vi "Main.vi"() -> ()   [LabVIEW 2020]
doc: "Este vi sirve para el control de monturas mecánicas y adquisición de datos de 2 instrumentos físicos.\n\nSolicitante:\nDr. Gabriel Ramos"
uses:
  <instrlib>/ZaberTSeries/Public/Utility/Request.ctl
  <instrlib>/ZaberTSeries/ZaberTSeries.lvlib
  Type Definitions/Datos a Guardar.ctl
  <vilib>/Utility/error.llb/DialogType.ctl
  <instrlib>/ZaberTSeries/Public/Utility/Response.ctl
  Type Definitions/Asistente de adquisicion Cluster.ctl
  <instrlib>/Stanford Research 830/Stanford Research 830.lvlib
  <instrlib>/Tektronix TDS 200 1000 2000 Series/Tektronix TDS 200 1000 2000 Series.lvlib
  Type Definitions/datos osciloscopio.ctl
  Type Definitions/Datos Zaber.ctl
  Type Definitions/parametros motores.ctl
  <instrlib>/Control de MaP/Control de MaP.lvlib
panel:
  out "Posición Actual":dbl[unit](slide) max=0.05
  in  "Stop Button":bool
  out "Datos":dbl[](graph)
  out "stop":bool
  out "Datos actuales":T1
  # "ENA"
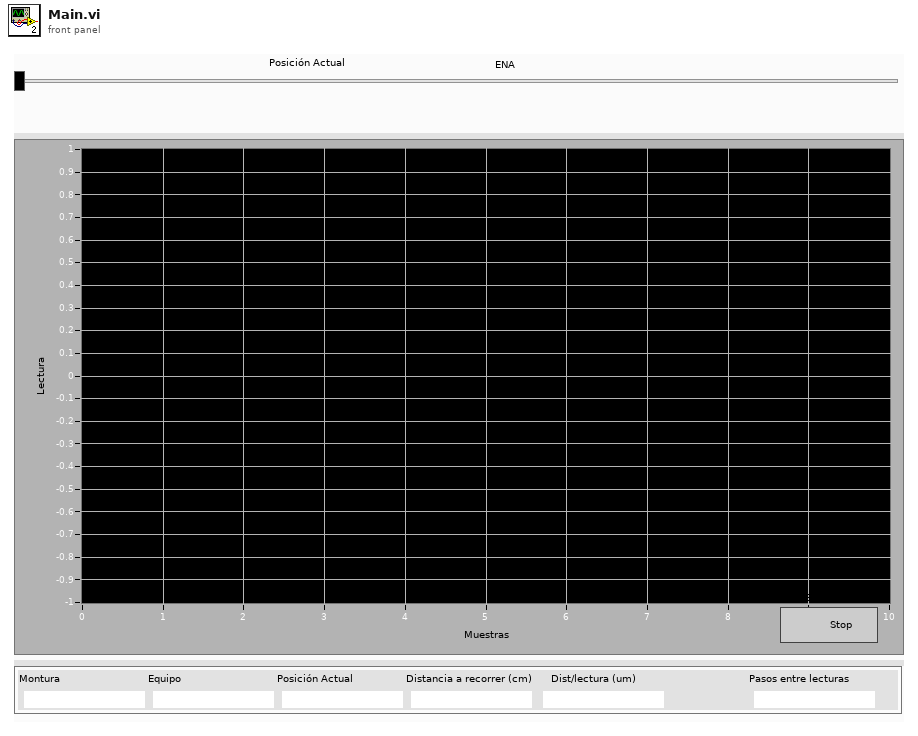
[diagram p1: front panel]
types:
  T1 = cluster{"Montura":string, "Equipo":string, "Posición Actual":string, "Distancia a recorrer (cm)":string, "Dist/lectura (um)":string, "Pasos entre lecturas":string}
  T2 = typedef "Asistente de adquisicion Cluster.ctl" = cluster{"Montura":enum16{"Zaber T-LSR450B", "Motor Bipolar", "Motor Unipolar"}, "Equipo a Utilizar":enum16{"SR830 Lock In", "TDS 2012B Osciloscope"}, "Datos Zaber":T3, "Datos Bipolar/Unipolar":T4, "Datos Archivo":cluster{"Ruta Archivo":path, "Nombre de Prueba":string}, "Datos actuales":cluster{"Montura":string, "Equipo":string, "Posición Actual":string, "Distancia Total a recorrer":string, "distancia Entre lecturas":string, "Pasos entre lecturas":string}, "Datos a Guardar In":T5, "Datos Osciloscopio":T6, "Datos Lock In":cluster{"Visa Lock in":refnum<visa-resource-name>}}
  T3 = typedef "Datos Zaber.ctl" = cluster{"Sentido de Adquisición":bool, "Comenzar Desde Home?":bool, "Distancia a recorrer (cm)":dbl, "Pasos motor":i32, "Distancia entre Lecturas (um)":dbl, "Puerto":refnum<visa-resource-name>}
  T4 = typedef "parametros motores.ctl" = cluster{"Puerto COM":refnum<visa-resource-name>, "Pasos entre Lecturas":u16, "Numero de lecturas":u32, "Sentido del motor":bool}
  T5 = typedef "Datos a Guardar.ctl" = cluster{"Datos Cursor Tektronix":string, "Datos Lokin":string, "Posición Cero":dbl[unit], "Posición Actual":dbl[unit]}
  T6 = typedef "datos osciloscopio.ctl" = cluster{"Sesión Visa Osciloscopio":refnum<visa-resource-name>, "Tipo de Adquisición":enum16{"Voltaje Pico Pico", "Voltaje RMS", "Cursor Tiempo"}, "Canal a Utilizar":enum16{"Canal 1", "Canal 2", "Canal 1 y 2"}, "Parametros de Adquisición":enum16{"Una Muestra", "Promedio"}, "Número Promedio":i32}
  T7 = typedef "ZaberTSeries.lvlib/Response.ctl" = cluster{"Device Number":u8, "Command":u8, "Data":i32}
  T8 = typedef "DialogType.ctl" = u16
  T9 = typedef "Constante estados proceso adquisición.ctl" = enum16{"Inicializar Equipo", "Inicializar Montura", "Leer Pos Actual", "Inicializar Archivo", "Leer Equipo", "guardar Archivo", "Mover Montura", "Corroborar distancias y Stop", "Cerrar Archivo y equipos"}
  T10 = typedef "ZaberTSeries.lvlib/Request.ctl" = cluster{"Device Number":u8, "Command":u8, "Data":i32, "Response Count":i32}
  T11 = enum16{"Zaber T-LSR450B", "Motor Bipolar", "Motor Unipolar"}
  T12 = cluster{"Montura":string, "Equipo":string, "Posición Actual":string, "Distancia Total a recorrer":string, "distancia Entre lecturas":string, "Pasos entre lecturas":string}
  T13 = enum32{"invalid app kind", "Development System", "Run Time System", "Student Edition", "Embedded LabVIEW", "Evaluation", "Custom"}
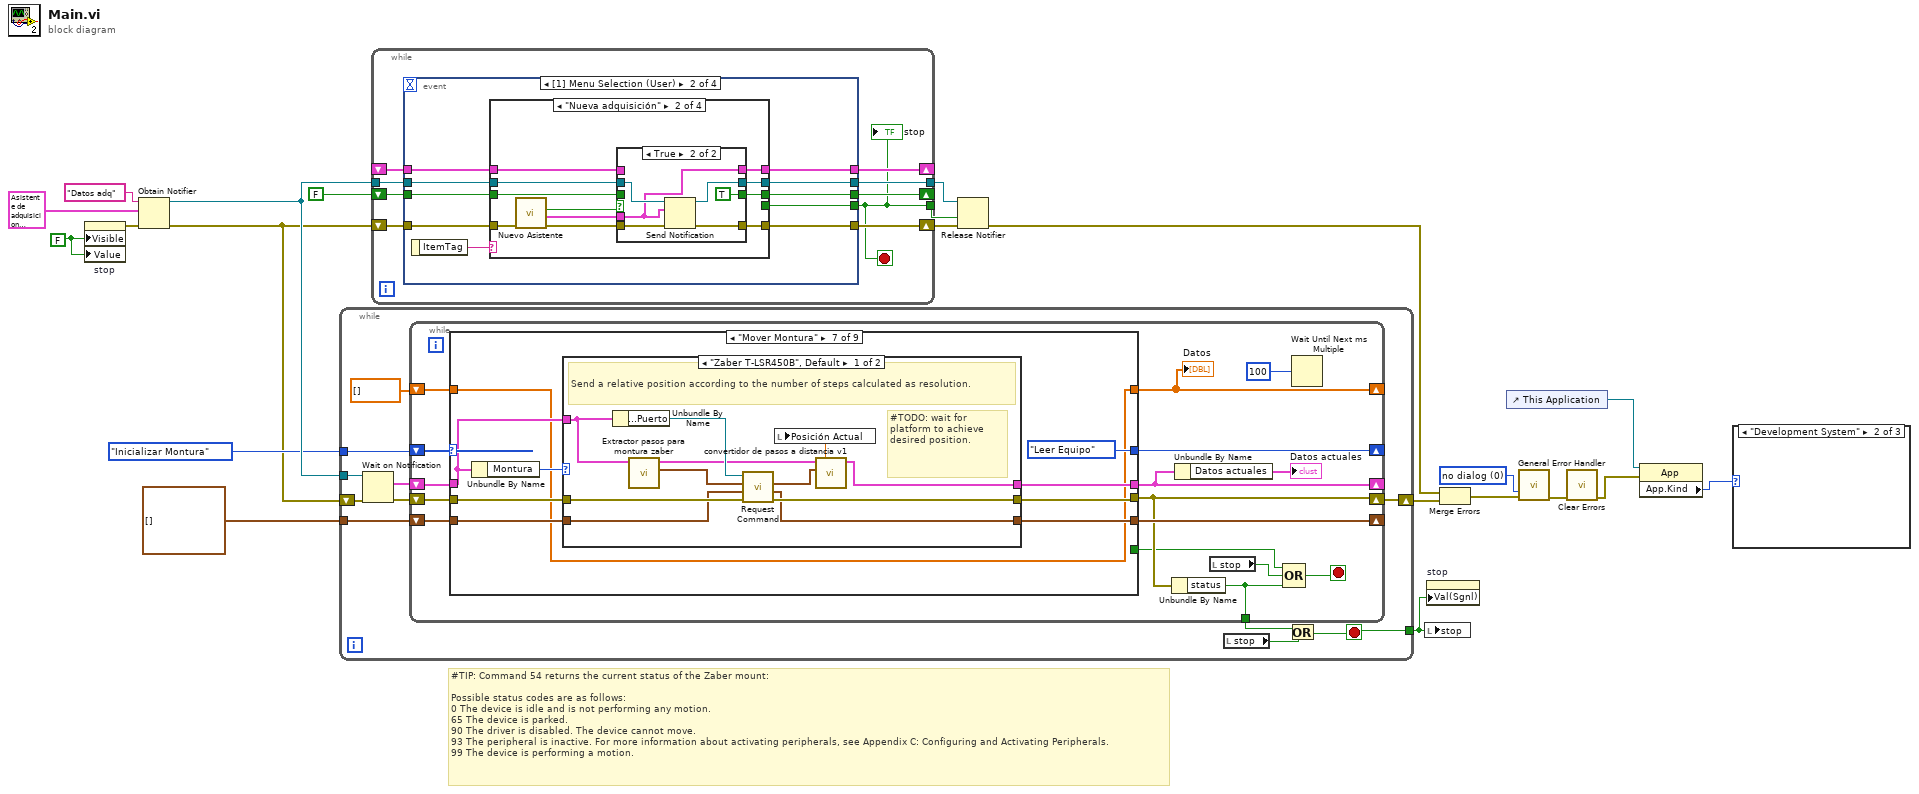
[diagram p0: block diagram]
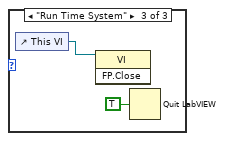
[diagram p3: hidden frame]
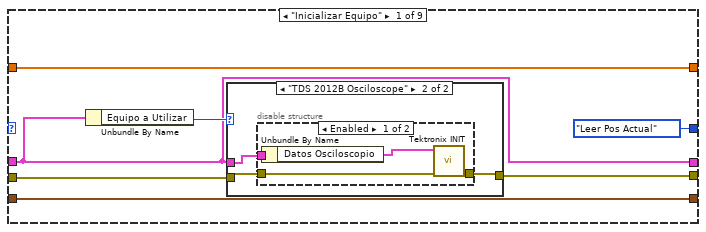
[diagram p4: hidden frame]
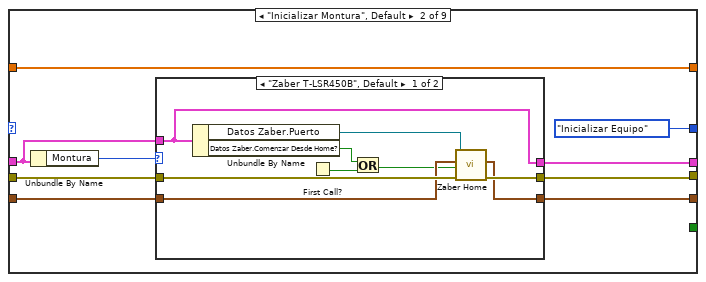
[diagram p7: hidden frame]
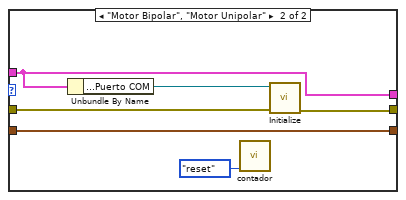
[diagram p8: hidden frame]
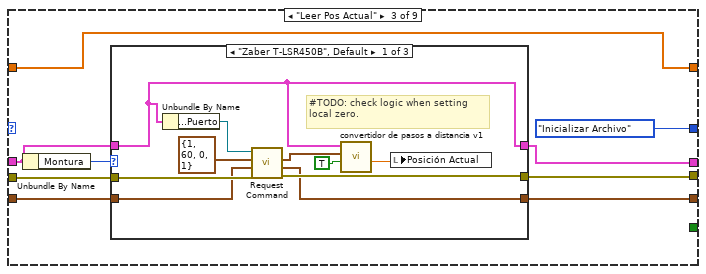
[diagram p9: hidden frame]
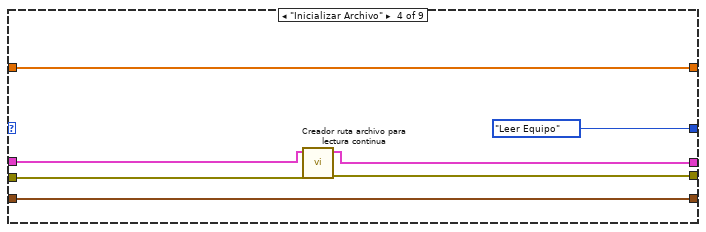
[diagram p12: hidden frame]
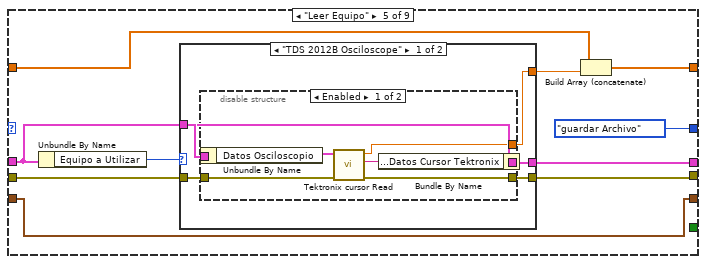
[diagram p13: hidden frame]
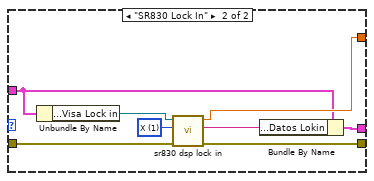
[diagram p15: hidden frame]
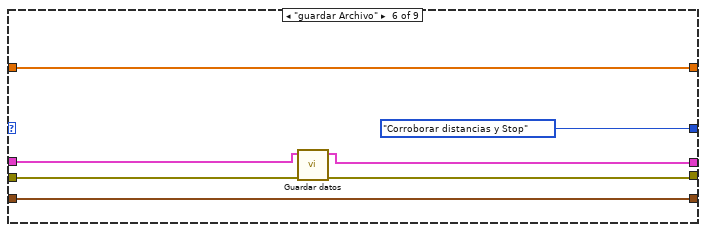
[diagram p16: hidden frame]
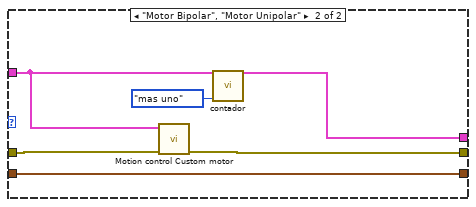
[diagram p17: hidden frame]
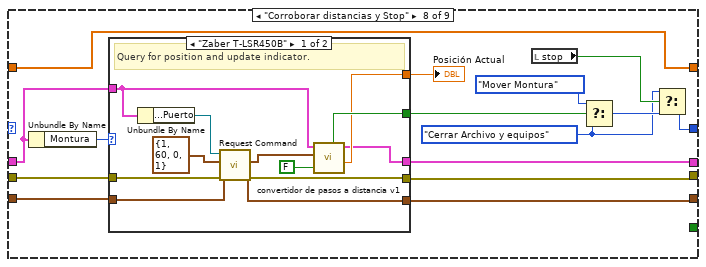
[diagram p18: hidden frame]
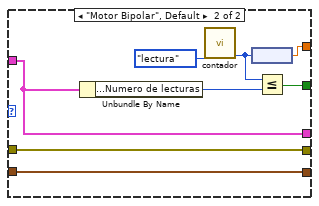
[diagram p19: hidden frame]
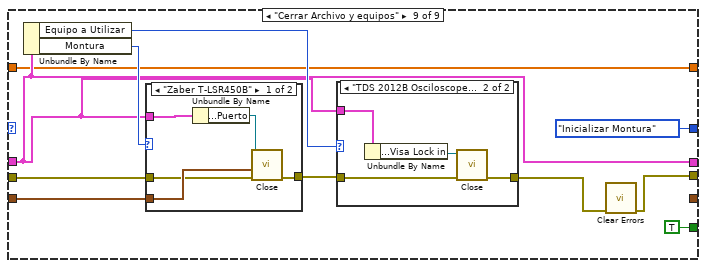
[diagram p20: hidden frame]
diagram:
  w2 = FALSE ("Visible")
  w12 = T8 0 items=["no dialog", "OK message", "continue or stop message", "OK message + warnings", "continue/stop + warnings"] ("type of dialog (OK msg:1)")
  # "#TIP: Command 54 returns the current status of the Zaber mount:\n\nPossible status codes are as follows:\n0 The device is idle and is not performing any motion.\n65 The device is parked.\n90 The driver is disabled. The device cannot move.\n93 The peripheral is inactive. For more information about activating peripherals, see Appendix C: Configuring and Activating Peripherals.\n99 The device is performing a motion."
  n1 = property on="stop" class="Bool (strict)"("Visible"=w2, "Value"=w2) -> (error out=w8:errorcluster)  [unwired: 2 in, 1 out]
  n2 = Obtain Notifier(name (unnamed)="Datos adq", notification data type=T2 {"Montura"=enum."Motor Bipolar", "Equipo a Utilizar"=enum."TDS 2012B Osciloscope", "Datos Zaber"={"Sentido de Adquisición"=FALSE, "Comenzar Desde Home?"=FALSE, "Distancia a recorrer (cm)"=0.0, "Pasos motor"=0, "Distancia entre Lecturas (um)"=0.0, "Puerto"=""}, "Datos Bipolar/Unipolar"={"Puerto COM"="", "Pasos entre Lecturas"=0, "Numero de lecturas"=0, "Sentido del motor"=TRUE}, "Datos Archivo"={"Ruta Archivo"=path "", "Nombre de Prueba"=""}, "Datos actuales"={"Montura"="", "Equipo"="", "Posición Actual"="", "Distancia Total a recorrer"="", "distancia Entre lecturas"="", "Pasos entre lecturas"=""}, "Datos a Guardar In"={"Datos Cursor Tektronix"="", "Datos Lokin"="", "Posición Cero"=0.0, "Posición Actual"=0.0}, "Datos Osciloscopio"={"Sesión Visa Osciloscopio"="Tektronix_TDS2012C", "Tipo de Adquisición"=enum."Voltaje Pico Pico", "Canal a Utilizar"=enum."Canal 1", "Parametros de Adquisición"=enum."Una Muestra", "Número Promedio"=2}, "Datos Lock In"={"Visa Lock in"="Tektronix_TDS2012C"}} ("Datos de Nueva Adquisición In"), error in (no error)=w8) -> (notifier out=w20:refnum<notifier>, error out=w11:errorcluster)  [unwired: 1 in, 1 out]
  n3 = while {
    tunnel: w20 -> [w32]
    shift-right: [w27] -> w15
    shift-left: w11 -> [w31]
    tunnel: Constante_estados_proceso_adquisición."Inicializar Montura" -> [w28]
    tunnel: T7[] [] ("Responses in") -> [w24]
    tunnel: [w23] -> w7
    stop <- w23 stop-if-true
    n4 = Wait on Notification(notifier=w32, error in (no error)=w31) -> (notification=w29:T2, error out=w30:errorcluster)  [unwired: 2 in, 2 out]
    n5 = while {
      shift-right: [w47] -> _
      shift-left: w28 -> [w48]
      shift-right: [w38] -> w27
      shift-left: w30 -> [w45]
      shift-right: [w39] -> _
      shift-left: w29 -> [w40]
      tunnel: [w35] -> w26
      shift-right: [w42] -> _
      shift-left: w24 -> [w43]
      shift-right: [w33] -> _
      shift-left: dbl[] [] -> [w34]
      stop <- w44 stop-if-true
      n6 = case shown="\"Mover Montura\"" w48 {
        tunnel: w40 -> [w52 w70 w93 w115 w127 w154 w164 w193 w224]
        tunnel: w45 -> [w51 w72 w96 w118 w129 w157 w166 w197 w226]
        tunnel: [w50 w71 w95 w117 w128 w156 w165 w196 w222] -> w38
        tunnel: [Constante_estados_proceso_adquisición."Leer Pos Actual" ("f") Constante_estados_proceso_adquisición."Inicializar Equipo" Constante_estados_proceso_adquisición."Inicializar Archivo" ("f") Constante_estados_proceso_adquisición."Leer Equipo" ("f") Constante_estados_proceso_adquisición."guardar Archivo" ("f") Constante_estados_proceso_adquisición."Corroborar distancias y Stop" ("f") Constante_estados_proceso_adquisición."Leer Equipo" ("f") w187 Constante_estados_proceso_adquisición."Inicializar Montura" ("f")] -> w47
        tunnel: [w52 w67 w90 w114 w124 w153 w161 w188 w224] -> w39
        tunnel: [_ _ _ _ _ _ _ _ TRUE ("stop")] -> w37
        tunnel: w43 -> [w49 w69 w92 w119 w125 w158 w163 w195 w227]
        tunnel: [w49 w68 w91 w119 w125 w158 w162 w194 _] -> w42
        tunnel: [w55 w66 w89 w116 w122 w155 w160 w186 w221] -> w33
        tunnel: w34 -> [w55 w66 w89 w116 w121 w155 w160 w186 w221]
        frame "Inicializar Equipo" {
          n7 = Unbundle By Name(w52) -> ("Equipo a Utilizar"=w53:enum16{"SR830 Lock In", "TDS 2012B Osciloscope"})
          n8 = case shown="\"TDS 2012B Osciloscope\"" w53 {
            tunnel: w52 -> [_ w59]
            tunnel: w51 -> [w56 w58]
            tunnel: [w56 w57] -> w50
            frame "SR830 Lock In", Default {
            }
            frame "TDS 2012B Osciloscope" {
              n9 = disable-structure shown="Enabled" {
                disable-tunnel: w59 -> [w63 _]
                disable-tunnel: w58 -> [w61 w64]
                disable-tunnel: [w60 w64] -> w57
                frame Enabled {
                  n10 = Unbundle By Name(w63) -> ("Datos Osciloscopio"=w62:T6)
                  n11 = call "Tektronix INIT.vi"("error in (no error)"=w61, "Datos Osciloscopio"=w62) -> ("error out"=w60:errorcluster)  [unwired: 9 in]
                }
                frame Disabled {
                }
              }
            }
          }
        }
        frame "Inicializar Montura", Default {
          n12 = Unbundle By Name(w70) -> ("Montura"=w73:T11)
          n13 = case shown="\"Zaber T-LSR450B\", Default" w73 {
            tunnel: w72 -> [w82 w86]
            tunnel: [w81 w85] -> w71
            tunnel: w70 -> [w78 w84]
            tunnel: w69 -> [w79 w88]
            tunnel: [w77 w88] -> w68
            tunnel: [w78 w84] -> w67
            frame "Zaber T-LSR450B", Default {
              n14 = Unbundle By Name(w78) -> ("Datos Zaber.Puerto"=w80:refnum<visa-resource-name>, "Datos Zaber.Comenzar Desde Home?"=w75:bool)
              n15 = First Call?() -> (First Call?: T/F=w76:bool)
              n16 = Or(x=w75, y=w76) -> (x .or. y?=w74:bool)
              n17 = call "Zaber Home.vi"("error in (no error)"=w82, "Ir a Home"=w74, "Responses in"=w79, "VISA Refnum in"=w80) -> ("error out"=w81:errorcluster, "Responses out"=w77:T7[])  [unwired: 5 in, 1 out]
            }
            frame "Motor Bipolar", "Motor Unipolar" {
              n18 = Unbundle By Name(w84) -> ("Datos Bipolar/Unipolar.Puerto COM"=w87:refnum<visa-resource-name>)
              n19 = call "contador.vi"("Opciones"=enum16{"reset", "mas uno", "lectura"}."reset") -> ()  [unwired: 10 in, 1 out]
              n20 = call <instrlib>:"Initialize.vi"("error in (no error)"=w86, "Puerto Serial"=w87) -> ("error out"=w85:errorcluster)  [unwired: 8 in, 1 out]
            }
          }
        }
        frame "Leer Pos Actual" {
          n21 = Unbundle By Name(w93) -> ("Montura"=w97:T11)
          n22 = case shown="\"Zaber T-LSR450B\", Default" w97 {
            tunnel: w96 -> [w107 w110 w113]
            tunnel: [w106 w110 w113] -> w95
            tunnel: w93 -> [w98 w108 w111]
            tunnel: w92 -> [w105 w109 w112]
            tunnel: [w104 w109 w112] -> w91
            tunnel: [w98 w108 w111] -> w90
            frame "Zaber T-LSR450B", Default {
              # "#TODO: check logic when setting local zero."
              n23 = Unbundle By Name(w98) -> ("Datos Zaber.Puerto"=w102:refnum<visa-resource-name>)
              n24 = call <instrlib>:"Request Command.vi"("error in (no error)"=w107, "Responses in"=w105, "Request"=T10 {"Device Number"=1, "Command"=60, "Data"=0, "Response Count"=1}, "VISA resource name"=w102) -> ("error out"=w106:errorcluster, "Responses out"=w104:T7[], "First Response"=w100:T7)  [unwired: 4 in, 1 out]
              n25 = call "convertidor de pasos a distancia v1.vi"("Set 0 vitual"=TRUE ("Inicializar"), "Respuesta Zaber"=w100, "Datos adquisición Input"=w98) -> ("Respuesta conversión zaber"=w103:dbl[unit])  [unwired: 6 in, 2 out]
              n26 = local write "Posición Actual"(w103) -> ()
            }
            frame "Motor Bipolar" {
            }
            frame "Motor Unipolar" {
            }
          }
        }
        frame "Inicializar Archivo" {
          n27 = call "Creador ruta archivo para lectura continua.vi"("error in (no error)"=w118, "Datos de Nueva Adquisición In"=w115) -> ("error out"=w117:errorcluster, "Datos de Nueva Adquisición out"=w114:T2)  [unwired: 4 in]
        }
        frame "Leer Equipo" {
          n28 = Unbundle By Name(w127) -> ("Equipo a Utilizar"=w130:enum16{"SR830 Lock In", "TDS 2012B Osciloscope"})
          n29 = case shown="\"TDS 2012B Osciloscope\"" w130 {
            tunnel: w127 -> [w133 w146]
            tunnel: w129 -> [w135 w151]
            tunnel: [w134 w150] -> w128
            tunnel: [w131 w147] -> w123
            tunnel: [w132 w145] -> w124
            frame "TDS 2012B Osciloscope" {
              n30 = disable-structure shown="Enabled" {
                disable-tunnel: w135 -> [w142 w143]
                disable-tunnel: [w141 w143] -> w134
                disable-tunnel: w133 -> [w140 w144]
                disable-tunnel: [w138 w144] -> w132
                disable-tunnel: [w136 _] -> w131
                frame Enabled {
                  n31 = Unbundle By Name(w140) -> ("Datos Osciloscopio"=w137:T6)
                  n32 = call "Tektronix cursor Read.vi"("error in (no error)"=w142, "Datos Osciloscopio"=w137) -> ("error out"=w141:errorcluster, "Dato"=w139:string, "CH1"=w136:dbl)  [unwired: 7 in]
                  n33 = Bundle By Name(cluster=w140, "Datos a Guardar In.Datos Cursor Tektronix"=w139) -> (w138:T2)
                }
                frame Disabled {
                }
              }
            }
            frame "SR830 Lock In" {
              w149 = u16 1 items=["X"=1, "Y"=2, "R"=3, "Theta"=4, "Channel 1"=5, "Channel 2"=6, "Aux In 1"=7, "Aux In 2"=8, "Aux In 3"=9, "Aux In 4"=10] ("Parameter (1: X)")
              n34 = Unbundle By Name(w146) -> ("Datos Lock In.Visa Lock in"=w152:refnum<visa-resource-name>)
              n35 = call "sr830 dsp lock in.vi"("error in (no error)"=w151, "Parameter (1: X)"=w149, "VISA resource name"=w152) -> ("error out"=w150:errorcluster, "Datos Lokin String"=w148:string, "Medición"=w147:dbl)  [unwired: 6 in]
              n36 = Bundle By Name(cluster=w146, "Datos a Guardar In.Datos Lokin"=w148) -> (w145:T2)
            }
          }
          n37 = Build Array (concatenate)(w121, w123) -> (w122:dbl[])
        }
        frame "guardar Archivo" {
          n38 = call "Guardar datos.vi"("error in"=w157, "Datos de Nueva Adquisición"=w154) -> ("error out"=w156:errorcluster, "Datos de Nueva Adquisición out"=w153:T2)  [unwired: 8 in]
        }
        frame "Mover Montura" {
          n39 = Unbundle By Name(w164) -> ("Montura"=w167:T11)
          n40 = case shown="\"Zaber T-LSR450B\", Default" w167 {
            tunnel: w166 -> [w179 w183]
            tunnel: [w178 w182] -> w165
            tunnel: w164 -> [w170 w181]
            tunnel: w163 -> [w176 w184]
            tunnel: [w175 w184] -> w162
            tunnel: [w169 w181] -> w161
            frame "Zaber T-LSR450B", Default {
              # "#TODO: wait for platform to achieve desired position."
              # "Send a relative position according to the number of steps calculated as resolution."
              n41 = Unbundle By Name(w170) -> ("Datos Zaber.Puerto"=w177:refnum<visa-resource-name>)
              n42 = call "Extractor pasos para montura zaber.vi"("Datos de Nueva Adquisición In"=w170) -> ("to Zaber"=w174:T10, "Datos de Nueva Adquisición Out"=w171:T2)  [unwired: 9 in]
              n43 = call <instrlib>:"Request Command.vi"("error in (no error)"=w179, "Responses in"=w176, "Request"=w174, "VISA resource name"=w177) -> ("error out"=w178:errorcluster, "Responses out"=w175:T7[], "First Response"=w173:T7)  [unwired: 4 in, 1 out]
              n44 = call "convertidor de pasos a distancia v1.vi"("Respuesta Zaber"=w173, "Datos adquisición Input"=w171) -> ("Respuesta conversión zaber"=w172:dbl[unit], "Datos adquisición Out"=w169:T2)  [unwired: 7 in, 1 out]
              n45 = local write "Posición Actual"(w172) -> ()
            }
            frame "Motor Bipolar", "Motor Unipolar" {
              n46 = call "Motion control Custom motor.vi"("error in (no error)"=w183, "Datos de Nueva Adquisición"=w181) -> ("error out"=w182:errorcluster)  [unwired: 9 in]
              n47 = call "contador.vi"("Opciones"=enum16{"reset", "mas uno", "lectura"}."mas uno") -> ()  [unwired: 10 in, 1 out]
            }
          }
        }
        frame "Corroborar distancias y Stop" {
          w189 = Constante_estados_proceso_adquisición."Cerrar Archivo y equipos" ("f")
          n48 = Unbundle By Name(w193) -> ("Montura"=w198:T11)
          n49 = case shown="\"Zaber T-LSR450B\"" w198 {
            tunnel: w197 -> [w210 w219]
            tunnel: [w209 w219] -> w196
            tunnel: w195 -> [w211 w218]
            tunnel: [w208 w218] -> w194
            tunnel: w193 -> [w200 w217]
            tunnel: [w207 w212] -> w192
            tunnel: [w201 w217] -> w188
            tunnel: [w206 w216] -> w185
            frame "Zaber T-LSR450B" {
              # "Query for position and update indicator."
              n50 = Unbundle By Name(w200) -> ("Datos Zaber.Puerto"=w205:refnum<visa-resource-name>)
              n51 = call <instrlib>:"Request Command.vi"("error in (no error)"=w210, "Responses in"=w211, "Request"=T10 {"Device Number"=1, "Command"=60, "Data"=0, "Response Count"=1}, "VISA resource name"=w205) -> ("error out"=w209:errorcluster, "Responses out"=w208:T7[], "First Response"=w203:T7)  [unwired: 4 in, 1 out]
              n52 = call "convertidor de pasos a distancia v1.vi"("Set 0 vitual"=FALSE ("Inicializar"), "Respuesta Zaber"=w203, "Datos adquisición Input"=w200) -> ("Respuesta conversión zaber"=w206:dbl[unit], "Datos adquisición Out"=w201:T2, "Seguir Moviendo"=w207:bool)  [unwired: 6 in]
            }
            frame "Motor Bipolar", Default {
              n53 = Unbundle By Name(w217) -> ("Datos Bipolar/Unipolar.Numero de lecturas"=w213:u32)
              n54 = call "contador.vi"("Opciones"=enum16{"reset", "mas uno", "lectura"}."lectura") -> ("Contador"=w214:i32)  [unwired: 10 in]
              n55 = node(w214) -> (w216:dbl[unit])
              n56 = Less Or Equal?(x=w214, y=w213) -> (x <= y?=w212:bool)
            }
          }
          "Posición Actual" <- w185
          n57 = local read "stop"() -> (w191:bool)
          n58 = Select(t=Constante_estados_proceso_adquisición."Mover Montura" ("f"), s=w192, f=w189) -> (s? t:f=w190:T9)
          n59 = Select(t=w189, s=w191, f=w190) -> (s? t:f=w187:T9)
        }
        frame "Cerrar Archivo y equipos" {
          n60 = Unbundle By Name(w224) -> ("Equipo a Utilizar"=w225:enum16{"SR830 Lock In", "TDS 2012B Osciloscope"}, "Montura"=w228:T11)
          n61 = case shown="\"Zaber T-LSR450B\"" w228 {
            tunnel: w227 -> [w243 _]
            tunnel: w226 -> [w242 w245]
            tunnel: [w241 w244] -> w223
            tunnel: w224 -> [w240 w246]
            frame "Zaber T-LSR450B" {
              n62 = Unbundle By Name(w240) -> ("Datos Zaber.Puerto"=w239:refnum<visa-resource-name>)
              n63 = call <instrlib>:"Close.vi"("error in (no error)"=w242, "Responses in"=w243, "VISA resource name"=w239) -> ("error out"=w241:errorcluster)  [unwired: 7 in, 1 out]
            }
            frame "Motor Unipolar", Default {
              n64 = disable-structure shown="Enabled" {
                disable-tunnel: w246 -> [w250 _]
                disable-tunnel: w245 -> [w248 w251]
                disable-tunnel: [w247 w251] -> w244
                frame Enabled {
                  n65 = Unbundle By Name(w250) -> ("Datos Bipolar/Unipolar.Puerto COM"=w249:refnum<visa-resource-name>)
                  n66 = call <instrlib>:"Close.vi"("error in (no error)"=w248, "VISA resource name"=w249) -> ("error out"=w247:errorcluster)  [unwired: 9 in]
                }
                frame Disabled {
                }
              }
            }
          }
          n67 = case shown="\"TDS 2012B Osciloscope\"" w225 {
            tunnel: w224 -> [w234 w238]
            tunnel: w223 -> [w232 w236]
            tunnel: [w231 w235] -> w220
            frame "SR830 Lock In", Default {
              n68 = Unbundle By Name(w234) -> ("Datos Lock In.Visa Lock in"=w233:refnum<visa-resource-name>)
              n69 = call <instrlib>:"Close.vi"("error in (no error)"=w232, "VISA resource name"=w233) -> ("error out"=w231:errorcluster)  [unwired: 9 in]
            }
            frame "TDS 2012B Osciloscope" {
              n70 = Unbundle By Name(w238) -> ("Datos Lock In.Visa Lock in"=w237:refnum<visa-resource-name>)
              n71 = call <instrlib>:"Close.vi"("error in (no error)"=w236, "VISA resource name"=w237) -> ("error out"=w235:errorcluster)  [unwired: 9 in]
            }
          }
          n72 = call <vilib>:"Clear Errors.vi"("error in (no error)"=w220) -> ("error out"=w222:errorcluster)  [unwired: 5 in, 1 out]
        }
      }
      "Datos" <- w33
      n73 = Unbundle By Name(w38) -> ("status"=w35:bool)
      n74 = Unbundle By Name(w39) -> ("Datos actuales"=→"Datos actuales":T12)
      n75 = local read "stop"() -> (w36:bool)
      n76 = Compound Arithmetic op=OR(w37, w36, w35) -> (w44:bool)
      n77 = Wait Until Next ms Multiple(millisecond multiple=u32 100) -> ()  [unwired: 1 out]
    }
    n78 = local read "stop"() -> (w25:bool)
    n79 = Or(x=w26, y=w25) -> (x .or. y?=w23:bool)
  }
  n80 = while {
    tunnel: w20 -> [w260]
    tunnel: [w258] -> w19
    tunnel: [w252] -> w17
    shift-right: [w257] -> w18
    shift-left: w11 -> [w259]
    shift-right: [w256] -> _
    shift-left: _ -> [w255]
    shift-right: [w253] -> _
    shift-left: FALSE -> [w254]
    stop <- w252 stop-if-true
    n81 = event shown="[1] Menu Selection (User)" {
      selector: _ -> [_ _ _ _]
      dyn-events: _ -> [_ _ _ _]
      timeout: _ -> [_ _ _ _]
      tunnel: w260 -> [w264 w274 w326 w330]
      tunnel: w259 -> [w263 w271 w323 w328]
      tunnel: [w264 w273 w326 w330] -> w258
      tunnel: [w263 w272 w323 w328] -> w257
      tunnel: [_ w267 w324 TRUE ("NewVal")] -> w252
      tunnel: [w262 w269 w327 w329] -> w256
      tunnel: w255 -> [w262 w268 w327 w329]
      tunnel: w254 -> [w261 w266 w325 w331]
      tunnel: [w261 w265 w325 w331] -> w253
      event Timeout {
        n82 = event-data() -> ()  [unwired: 1 in, 2 out]
      }
      event Menu Selection (User) {
        n83 = event-data() -> ("ItemTag"=w270:string)  [unwired: 1 in]
        n84 = case shown="\"Nueva adquisición\"" w270 {
          tunnel: w274 -> [w279 w303 w316 w321]
          tunnel: [w280 w302 w316 w321] -> w273
          tunnel: [w281 w301 w314 w320] -> w272
          tunnel: w271 -> [w282 w293 w314 w320]
          tunnel: [w276 w295 w317 w322] -> w269
          tunnel: w268 -> [w278 w294 w317 w322]
          tunnel: [_ _ _ TRUE] -> w267
          tunnel: w266 -> [w277 w297 w315 w318]
          tunnel: [w275 w298 w315 w318] -> w265
          frame "Repetir Adquisición", Default {
            n85 = case shown="True" w277 {
              selector: w277 -> [w283 w288]
              tunnel: w282 -> [w285 w292]
              tunnel: [w285 w291] -> w281
              tunnel: [w286 w290] -> w280
              tunnel: w279 -> [w286 w289]
              tunnel: w278 -> [w284 w287]
              tunnel: [w284 w287] -> w276
              tunnel: [w283 w288] -> w275
              frame False {
              }
              frame True {
                n86 = Send Notification(notification=w287, notifier=w289, error in (no error)=w292) -> (notifier out=w290:refnum<notifier>, error out=w291:errorcluster)
              }
            }
          }
          frame "Nueva adquisición" {
            n87 = call "Nuevo Asistente.vi"("error in (no error)"=w293) -> ("error out"=w299:errorcluster, "Datos de Nueva Adquisición"=w296:T2, "Iniciar Prueba"=w300:bool)  [unwired: 8 in]
            n88 = case shown="True" w300 {
              tunnel: w303 -> [w307 w310]
              tunnel: w299 -> [w306 w313]
              tunnel: [w307 w312] -> w302
              tunnel: [w306 w311] -> w301
              tunnel: [w305 TRUE] -> w298
              tunnel: w297 -> [w305 _]
              tunnel: w296 -> [_ w308]
              tunnel: [w304 w308] -> w295
              tunnel: w294 -> [w304 _]
              frame False {
              }
              frame True {
                n89 = Send Notification(notification=w308, notifier=w310, error in (no error)=w313) -> (notifier out=w312:refnum<notifier>, error out=w311:errorcluster)
              }
            }
          }
          frame "Osciloscopio en Tiempo Real" {
            n90 = call "Tektronix TDS 200 1000 2000 Series Acquire Continuous Waveform.vi"() -> ()  [unwired: 1 in]
          }
          frame "Salir" {
          }
        }
      }
      event "stop": Value Change {
        n91 = event-data() -> ("NewVal"=w324:bool)  [unwired: 1 in]
      }
      event "Stop Button": Value Change {
        n92 = event-data() -> ()  [unwired: 1 in, 1 out]
      }
    }
    "stop" <- w252
  }
  n93 = Release Notifier(notifier=w19, force destroy? (F)=w17, error in (no error)=w18) -> (error out=w14:errorcluster)  [unwired: 2 out]
  n94 = local write "stop"(w7) -> ()
  n95 = property on="stop" class="Bool (strict)"("Val(Sgnl)"=w7) -> ()  [unwired: 2 in, 2 out]
  n96 = Merge Errors(w14, w15) -> (w13:errorcluster)
  n97 = control-ref of="This Application"() -> (w6:refnum<vi>)
  n98 = call <vilib>:"General Error Handler.vi"("type of dialog (OK msg:1)"=w12, "error in (no error)"=w13) -> ("error out"=w5:errorcluster)  [unwired: 9 in, 4 out]
  n99 = call <vilib>:"Clear Errors.vi"("error in (no error)"=w5) -> ("error out"=w4:errorcluster)  [unwired: 5 in, 1 out]
  n100 = property class="App"(reference=w6, error in=w4) -> ("App.Kind"=w3:T13)  [unwired: 2 out]
  n101 = case shown="\"Development System\"" w3 {
    frame "invalid app kind", Default {
    }
    frame "Development System" {
    }
    frame "Run Time System" {
      n102 = control-ref of="This VI"() -> (w334:refnum<vi>)
      n103 = invoke class="VI" method="FP.Close"(reference=w334) -> ()  [unwired: 2 in, 3 out]
      n104 = Quit LabVIEW(quit? (T)=TRUE) -> ()
    }
  }
